vi "ReturnFENRows.vi"(8 "error in (no error)":errorcluster, 11 "Board in":refnum<class "Board.lvclass">) -> (0 "error out":errorcluster, 2 "StandardPieceLocation":string[](array[string]), 3 "Board out":refnum<class "Board.lvclass">)   [LabVIEW 2020, in "Board.lvclass"]
doc: "builds the piece location by ROW of board"
uses:
  Board.lvclass
  Board.lvclass/Board.ctl
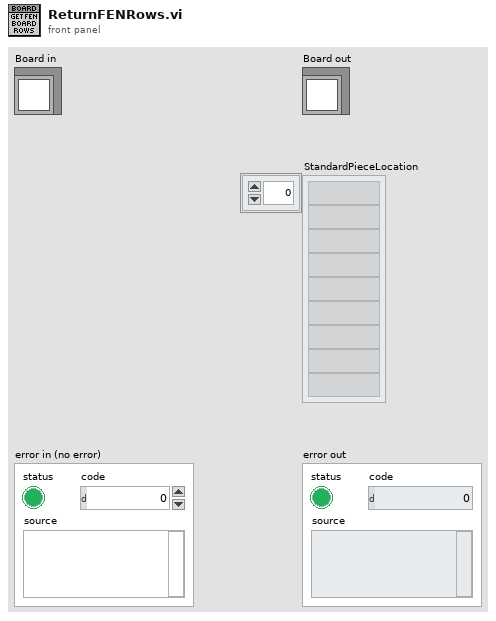
[diagram p1: front panel]
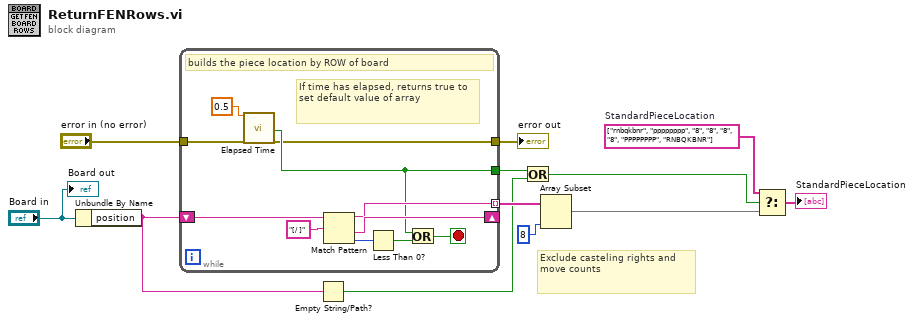
[diagram p0: block diagram]
diagram:
  w8 = string[] ["rnbqkbnr", "pppppppp", "8", "8", "8", "8", "PPPPPPPP", "RNBQKBNR"]  # StandardPieceLocation
  # "Exclude casteling rights and move counts"
  n1 = Unbundle By Name("Board in") -> ("position"=w10:string)
  n2 = while {
    shift-right: [w21] -> _
    shift-left: w10 -> [w16]
    tunnel: [w20] -> w4 mode=indexing
    tunnel: [w17] -> w9
    tunnel: [w13] -> w12
    tunnel: "error in (no error)" -> [w14]
    stop <- w18 stop-if-true
    # "If time has elapsed, returns true to set default value of array"
    # "builds the piece location by ROW of board"
    n3 = call "Elapsed Time"("Time Target (s)"=0.5, "error in (no error)"=w14) -> ("Time has Elapsed"=w17:bool, "error out"=w13:errorcluster)  [unwired: 10 in, 6 out]
    n4 = Match Pattern(string=w16, regular expression="[/ ]") -> (before substring=w20:string, after substring=w21:string, offset past match=w23:i32)  [unwired: 1 in, 1 out]
    n5 = Less Than 0?(x=w23) -> (x < 0?=w15:bool)
    n6 = Or(x=w17, y=w15) -> (x .or. y?=w18:bool)
  }
  "error out" <- w12
  n7 = Empty String/Path?(string/path=w10) -> (empty?=w1:bool)
  n8 = Or(x=w9, y=w1) -> (x .or. y?=w2:bool)
  n9 = Array Subset(array=w4, length=8) -> (w7:string[])  [unwired: 1 in]
  n10 = Select(t=w8, s=w2, f=w7) -> (s? t:f=→"StandardPieceLocation":string[])
  "Board out" <- "Board in"
